vi "gfitsio-write-column-u8-1d.vi"(4 "units":string, 6 "row":i32, 7 "column":string, 8 "error in (no error)":errorcluster, 9 "data":u8[](array[numeric]), 10 "variable length? (T:yes)":bool=TRUE, 11 "gfits refnum":T1) -> (0 "error out":errorcluster, 3 "dup gfits refnum":T1)   [LabVIEW 2024, in "gfitsio.lvlib"]
doc: "This VI is not compatible with ASCII tables.\n\nWrite data to the table column (doing data type conversion if necessary). If the column does not exist, it is created using the parameters specified to this VI. If the row in which this data will be added does not exist it is appended to the table. If the row does exist then the cell is overwritten.\n\nThe FITS Standard recommends that only letters, digits, and the underscore character be used in column names (the ttype parameter) with no embedded spaces. Trailing blank characters are not significant. It is recommended that all the column names in a given table be unique within the first 8 characters, and strongly recommended that the names be unique within the first 16 characters.\n\nPhysical units are asscociated with the data in this column. GFITSIO writes this string to the FITS file the first time data is written to the column. If different units are supplied on a subsequent write GFITSIO will not overwrite the existing units."
uses:
  gfitsio.lvlib
  gfitsio-refnum.ctl
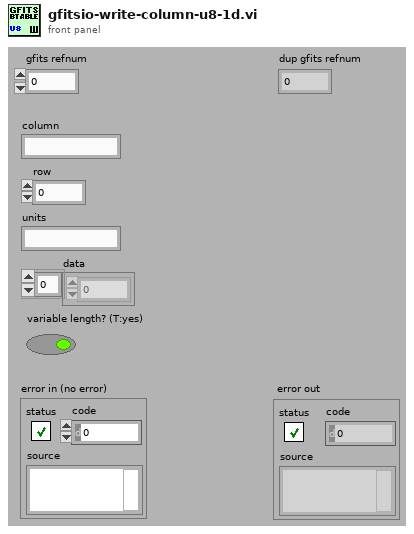
[diagram p1: front panel]
types:
  T1 = typedef "gfitsio.lvlib/gfitsio-refnum.ctl" = u64
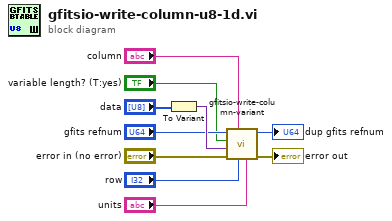
[diagram p0: block diagram]
diagram:
  n1 = To Variant(anything="data") -> (Variant=w10:variant)
  n2 = call "gfitsio-write-column-variant.vi"("units"="units", "row"="row", "column"="column", "error in (no error)"="error in (no error)", "data"=w10, "Variable Size? (F)"="variable length? (T:yes)", "gfits refnum"="gfits refnum") -> ("error out"=→"error out":errorcluster, "dup gfits refnum"=→"dup gfits refnum":T1)  [unwired: 3 in]
